vi "Add Required Status Channels.vi"(8 "error in":errorcluster, 11 "custom device reference":T1 format="%.0x") -> (0 "error out":errorcluster, 2 "status section ref out":T1 format="%.0x", 3 "custom device reference out":T1 format="%.0x")   [LabVIEW 2020, in "Ballard ARINC 429 Scripting.lvlib"]
doc: "Adds 'Status' section and required channels including error status channels and asynchronous loop time."
uses:
  Ballard ARINC 429 Scripting.lvlib
  <vilib>/NI VeriStand/Custom Device API/Custom Device Item Ref.ctl
  <vilib>/NI VeriStand/Custom Device API/Custom Device API.lvlib
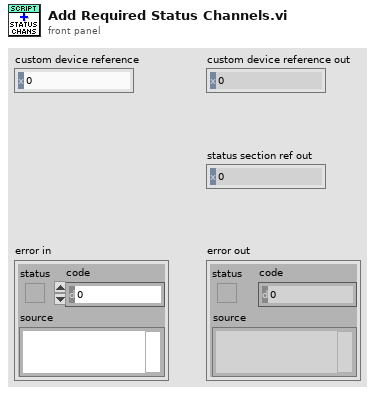
[diagram p1: front panel]
types:
  T1 = typedef "Custom Device API.lvlib/Custom Device Item Ref.ctl" = u64
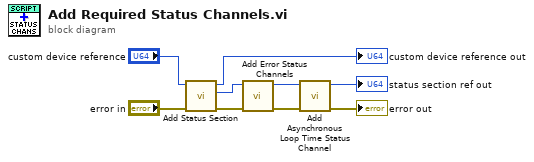
[diagram p0: block diagram]
diagram:
  n1 = call "Add Status Section.vi"("error in"="error in", "custom device ref"="custom device reference") -> ("error out"=w6:errorcluster, "status ref"=w9:T1, "custom device ref out"=→"custom device reference out":T1)  [unwired: 7 in]
  n2 = call "Add Error Status Channels.vi"("error in"=w6, "status section ref"=w9) -> ("error out"=w8:errorcluster, "status section ref out"=w7:T1)  [unwired: 8 in]
  n3 = call "Add Asynchronous Loop Time Status Channel.vi"("error in"=w8, "status section ref"=w7) -> ("error out"=→"error out":errorcluster, "status section ref out"=→"status section ref out":T1)  [unwired: 8 in]
